vi "PH_Stepmotor_BaseClass.get Axis Attributes.vi"(0 "VI in":refnum<vi>, 2 "Axis":i32=-1, 5 "error in (no error)":errorcluster) -> (14 "VI out":refnum<vi>, 16 "Axis found?":bool, 17 "Axis Attributes":T1, 19 "error out":errorcluster)   [LabVIEW 2014, in "PH_Stepmotor_BaseClass.lvlib"]
uses:
  PH_Stepmotor_BaseClass.lvlib
  PH_Stepmotor_BaseClass.Axis Attributes.ctl
  PH_Stepmotor_BaseClass.Axis Settings.ctl
  PH_Stepmotor_BaseClass.Motor Type.ctl
  PH_Stepmotor_BaseClass.Axis DIM Service IDs.ctl
  PH_Stepmotor_BaseClass.Axis Activity.ctl
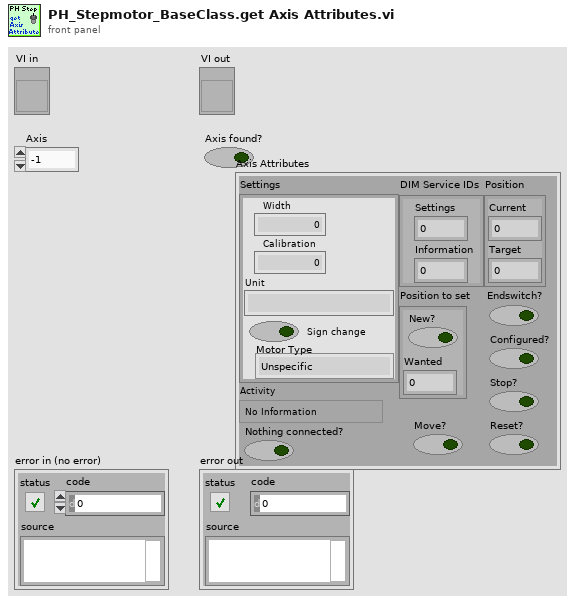
[diagram p1: front panel]
types:
  T1 = typedef "PH_Stepmotor_BaseClass.lvlib/PH_Stepmotor_BaseClass.Axis Attributes.ctl" = cluster{"Settings":T2, "Endswitch?":bool, "DIM Service IDs":T4, "Activity":T5, "Configured?":bool, "Position":cluster{"Current":i32, "Target":i32}, "Position to set":cluster{"New?":bool, "Wanted":i32}, "Stop?":bool, "Reset?":bool, "Move?":bool, "Nothing connected?":bool}
  T2 = typedef "PH_Stepmotor_BaseClass.lvlib/PH_Stepmotor_BaseClass.Axis Settings.ctl" = cluster{"Sign change":bool, "Width":dbl, "Calibration":dbl, "Unit":string, "Motor Type":T3, "Unit Width":string, "Unit CF":string}
  T3 = typedef "PH_Stepmotor_BaseClass.lvlib/PH_Stepmotor_BaseClass.Motor Type.ctl" = enum16{"Unspecific", "OWIS 49.120.2633", "OWIS 49.060.1033", "OWIS 43.040.2558", "Diamond Motion 2200 series", "OWIS 49.120.266B.MV6", "Calorimeter", "Linear Stage 1", "MICOS VT-80", "MICOS VT-80 S", "Standa Rotstage nt0.95A", "PUF RA 320.200", "PUF RA 800.200", "PUF RA 800.400", "PUF RA 400.50", "1324.nn.800.50", "1324.n9c.800.50", "1324.nn.320.200", "1324.nn.400.200", "1324.nn.800.200", "1324.nn.400.50", "1324.8c9c.800.50", "1324.8c9c.400.200"}
  T4 = typedef "PH_Stepmotor_BaseClass.lvlib/PH_Stepmotor_BaseClass.Axis DIM Service IDs.ctl" = cluster{"Settings":i32, "Information":i32}
  T5 = typedef "PH_Stepmotor_BaseClass.lvlib/PH_Stepmotor_BaseClass.Axis Activity.ctl" = enum16{"No Information", "stopped", "running", "Failure", "Alarm", "stopped at backward ES", "stopped at foreward ES"}
  T6 = typedef "PH_Stepmotor_BaseClass.lvlib/PH_Stepmotor_BaseClass.i attribute.ctl" = cluster{"Device Error":errorcluster, "Axes PSDB Thread":cluster{"Ref":refnum<vi>, "Q-Ref":refnum<queue>, "Data Status":T7}, "Axes":T1[], "Axes PSDB Infos":cluster{"GUI Name":string, "PSDB Instance ID":i32, "PSDB Status Service ID":i32, "Axis":i32, "Class":string}[], "GUI Refs":T8}
  T7 = typedef "PH_PSDBWriter.lvlib/PH_PSDBWriter.Data Status.ctl" = i16
  T8 = typedef "PH_Stepmotor_BaseClass.lvlib/PH_Stepmotor_BaseClass.GUI Refs.ctl" = cluster{"Axes Configuration":refnum<vi>, "Device Error":refnum<vi>, "Axes PSDB Infos":refnum<vi>}
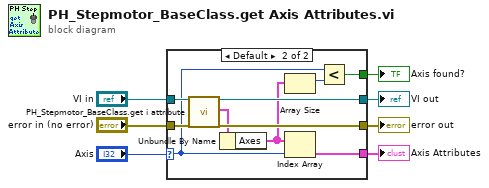
[diagram p0: block diagram]
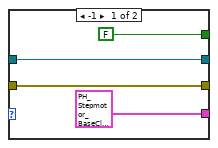
[diagram p2: hidden frame]
diagram:
  n1 = case shown="Default" "Axis" {
    selector: "Axis" -> [_ w14]
    tunnel: "error in (no error)" -> [w10 w21]
    tunnel: [w10 w20] -> w2
    tunnel: "VI in" -> [w11 w19]
    tunnel: [w11 w18] -> w4
    tunnel: [T1 {"Settings"={"Sign change"=FALSE, "Width"=0.0, "Calibration"=0.0, "Unit"="", "Motor Type"=enum."Unspecific", "Unit Width"="", "Unit CF"=""}, "Endswitch?"=FALSE, "DIM Service IDs"={"Settings"=0, "Information"=0}, "Activity"=enum."No Information", "Configured?"=FALSE, "Position"={"Current"=0, "Target"=0}, "Position to set"={"New?"=FALSE, "Wanted"=0}, "Stop?"=FALSE, "Reset?"=FALSE, "Move?"=FALSE, "Nothing connected?"=FALSE} ("motor") w16] -> w6
    tunnel: [FALSE w12] -> w7
    frame -1 {
    }
    frame Default {
      n2 = call "PH_Stepmotor_BaseClass.get i attribute.vi"("i ref in"=w19, "error in (no error)"=w21) -> ("i ref out"=w18:refnum<vi>, "i attribute"=w17:T6, "error out"=w20:errorcluster)  [unwired: 15 in]
      n3 = Unbundle By Name(w17) -> ("Axes"=w15:T1[])
      n4 = Array Size(array=w15) -> (size(s)=w13:i32)
      n5 = Index Array(array=w15, index=w14) -> (element=w16:T1)
      n6 = Less?(x=w14, y=w13) -> (x < y?=w12:bool)
    }
  }
  "Axis found?" <- w7
  "Axis Attributes" <- w6
  "VI out" <- w4
  "error out" <- w2
